vi "ReportElementCount.vi"(1 "Destination":T1={"Subsystem Id"=90, "Node Id"=1, "Component Id"=1}, 2 "Source":T1={"Subsystem Id"=3, "Node Id"=1, "Component Id"=1}) -> (0 "Encoded JAUS Message":string)   [LabVIEW 2009]
uses:
  Support Files/Address.ctl
panel:
  in  "Command Code":string="D\u001c"
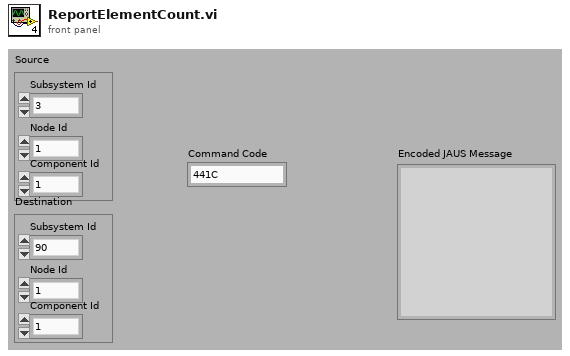
[diagram p1: front panel]
types:
  T1 = typedef "Address.ctl" = cluster{"Subsystem Id":u16, "Node Id":u8, "Component Id":u8}
  T2 = cluster{"unsigned byte array[0]":u8, "unsigned byte array[1]":u8}
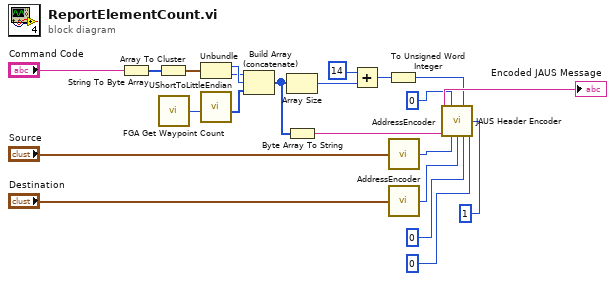
[diagram p0: block diagram]
diagram:
  n1 = String To Byte Array(string="Command Code") -> (unsigned byte array=w9:u8[])
  n2 = Array To Cluster(array=w9) -> (cluster=w8:T2)
  n3 = call "FGA Get Waypoint Count.vi"() -> ("count"=w2:u16)
  n4 = Unbundle(w8) -> ("unsigned byte array[0]"=w7:u8, "unsigned byte array[1]"=w6:u8)
  n5 = call "UShortToLittleEndian.vi"("Number"=w2) -> ("byte array"=w1:u8[])  [unwired: 10 in]
  n6 = Build Array (concatenate)(w6, w7, w1) -> (w13:u8[])
  n7 = Array Size(array=w13) -> (size(s)=w11:i32)
  n8 = Byte Array To String(unsigned byte array=w13) -> (string=w15:string)
  n9 = Add(x=14, y=w11) -> (x+y=w10:i32)
  n10 = To Unsigned Word Integer(number=w10) -> (unsigned 16bit integer=w3:u16)
  n11 = call "AddressEncoder.vi"("Address Cluster"="Source") -> ("Address"=w21:u32)
  n12 = call "AddressEncoder.vi"("Address Cluster"="Destination") -> ("Address"=w20:u32)
  n13 = call "JAUS Header Encoder.vi"("Message Type (0-5)"=u8 0, "Data Size (8-23)"=w3, "Priority(40-41)"=u8 1, "Payload"=w15, "Source ID (80-95)"=w21, "Destination ID (48-79)"=w20, "Data Flags (46-47)"=u8 0, "Ack/Nak (44-45)"=u8 0) -> ("Encoded JAUS Message"=→"Encoded JAUS Message":string)  [unwired: 7 in]
